vi "NodifyROS.vi"(1 "ROS in":T1) -> (0 "ROS out":T1)   [LabVIEW 2012]
uses:
  <userlib>/ROSforLV/ROS/Code/SubVIs/_ROSControl.ctl
  <userlib>/ROSforLV/ROS/Code/SubVIs/_ROSDirection.ctl
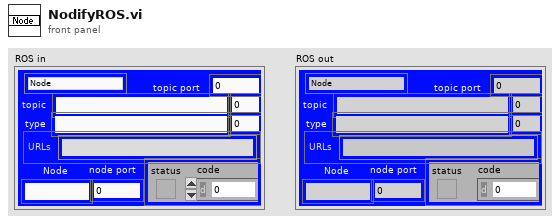
[diagram p1: front panel]
types:
  T1 = typedef "_ROSControl.ctl" = cluster{"topic port":u16, "Node":string, "topic":string, "type":string, "node port":u16, "error ":errorcluster, "Direction":T2, "APIs":string[], "Update (ms)":u16, "write queue":u16}
  T2 = typedef "_ROSDirection.ctl" = enum16{"Node", "Publisher", "Subscriber", "Service Client"}
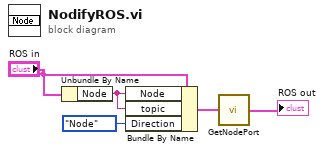
[diagram p0: block diagram]
diagram:
  n1 = Unbundle By Name("ROS in") -> ("Node"=w3:string)
  n2 = Bundle By Name(cluster="ROS in", "Node"=w3, "topic"=w3, "Direction"=_ROSDirection."Node") -> (w2:T1)
  n3 = call <userlib>:"GetNodePort.vi"("ROS in"=w2) -> ("ROS out"=→"ROS out":T1)
